vi "read status string.vi"(0 "VISA resource name":refnum<visa-resource-name>="GPIB0::12::INSTR", 1 "error in (no error)":errorcluster) -> (2 "VISA resource name out":refnum<visa-resource-name>, 3 "Mode":u16(ring) items=["SLEEP", "WARM-UP", "STANDBY", "OPERATE", "FAULT"], 4 "error out":errorcluster)   [LabVIEW 2017, in "MicrowaveAmplifier.lvlib"]
uses:
  MicrowaveAmplifier.lvlib
panel:
  out "read buffer":string
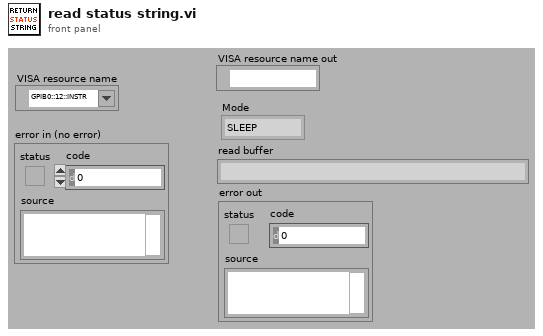
[diagram p1: front panel]
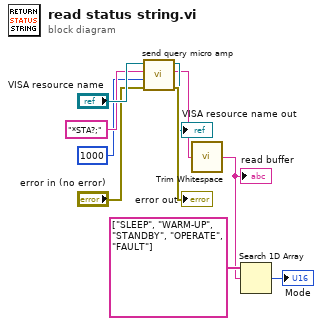
[diagram p0: block diagram]
diagram:
  n1 = call "send query micro amp.vi"("error in (no error)"="error in (no error)", "Bytes Count"=u32 1000 ("bytes to read (1000) 2"), "write buffer"="*STA?;" ("write buffer 2"), "VISA resource name"="VISA resource name") -> ("error out"=→"error out":errorcluster, "read buffer"=w1:string, "VISA resource name out"=→"VISA resource name out":refnum<visa-resource-name>)  [unwired: 5 in]
  n2 = call <vilib>:"Trim Whitespace.vi"("string"=w1) -> ("trimmed string"=w9:string)  [unwired: 1 in]
  "read buffer" <- w9
  n3 = Search 1D Array(1D array=string[] ["SLEEP", "WARM-UP", "STANDBY", "OPERATE", "FAULT"], element=w9) -> (index of element=→"Mode":i32)  [unwired: 1 in]
